vi "Add Test Case.vi"(10 "Test Case to add":refnum<class "LUnit Test Case.lvclass">, 11 "Test Suite In":refnum<class "LUnit Test Suite.lvclass">) -> (3 "Test Suite Out":refnum<class "LUnit Test Suite.lvclass">)   [LabVIEW 2020, in "LUnit Test Suite.lvclass"]
uses:
  LUnit Test Suite.lvclass
  Test Case/LUnit Test Case.lvclass
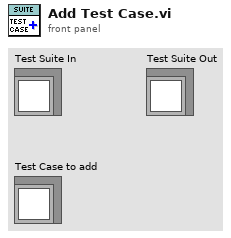
[diagram p1: front panel]
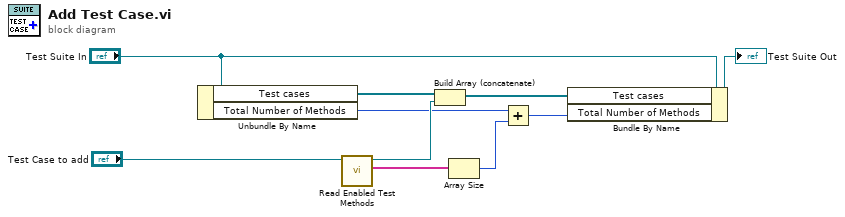
[diagram p0: block diagram]
diagram:
  n1 = Unbundle By Name("Test Suite In") -> ("Test cases"=w9:refnum<class "LUnit Test Case.lvclass">[], "Total Number of Methods"=w3:i32)
  n2 = call "Read Enabled Test Methods.vi"("LUnit Test Case In"="Test Case to add") -> ("Names"=w4:string[], "LUnit Test Case Out"=w5:refnum<class "LUnit Test Case.lvclass">)  [unwired: 8 in, 1 out]
  n3 = Build Array (concatenate)(w9, w5) -> (w7:refnum<class "LUnit Test Case.lvclass">[])
  n4 = Array Size(array=w4) -> (size(s)=w2:i32)
  n5 = Add(x=w3, y=w2) -> (x+y=w1:i32)
  n6 = Bundle By Name(cluster="Test Suite In", "Test cases"=w7, "Total Number of Methods"=w1) -> (→"Test Suite Out":refnum<class "LUnit Test Suite.lvclass">)
